vi "Save Last Print.vi"(8 "error in (no error)":errorcluster, 9 "Printing Date":string, 10 "SN":u32, 11 "Part Name":string) -> (0 "error out":errorcluster)   [LabVIEW 2017]
uses:
  <vilib>/Utility/config.llb/Write Key (U32).vi
  <vilib>/Utility/config.llb/Write Key (String).vi
  <vilib>/Utility/config.llb/NI_LVConfig.lvlib
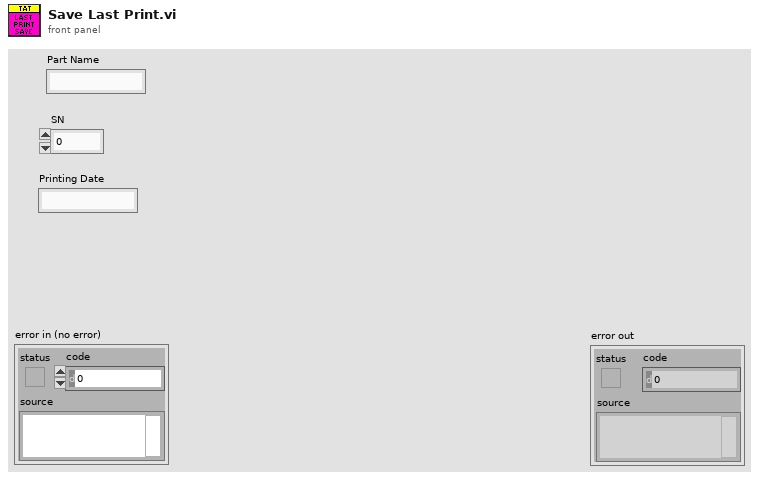
[diagram p1: front panel]
types:
  T1 = enum32{"invalid app kind", "Development System", "Run Time System", "Student Edition", "Embedded LabVIEW", "Evaluation", "Custom"}
  T2 = typedef "NI_LVConfig.lvlib/Config Data RefNum.ctl" = refnum<k1>
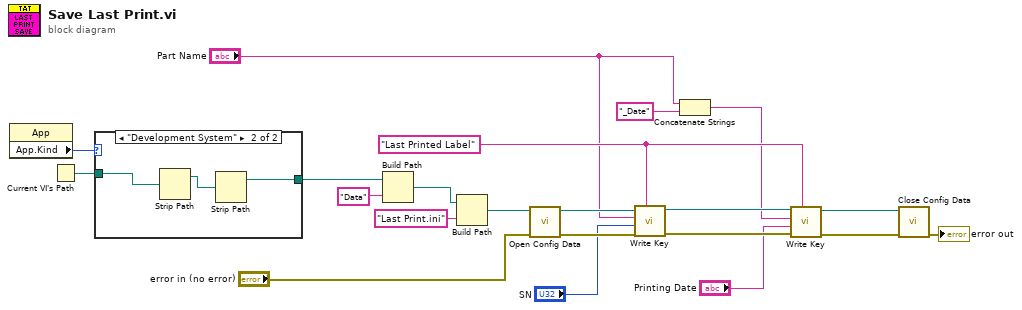
[diagram p0: block diagram]
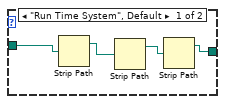
[diagram p2: hidden frame]
diagram:
  w7 = "Last Printed Label" ("section")
  n1 = property class="App"() -> ("App.Kind"=w20:T1)  [unwired: 2 in, 2 out]
  n2 = Current VI's Path() -> (path=w21:path)
  n3 = case shown="\"Development System\"" w20 {
    tunnel: w21 -> [w23 w27]
    tunnel: [w22 w26] -> w15
    frame "Run Time System", Default {
      n4 = Strip Path(path=w23) -> (stripped path=w25:path)  [unwired: 1 out]
      n5 = Strip Path(path=w25) -> (stripped path=w24:path)  [unwired: 1 out]
      n6 = Strip Path(path=w24) -> (stripped path=w22:path)  [unwired: 1 out]
    }
    frame "Development System" {
      n7 = Strip Path(path=w27) -> (stripped path=w28:path)  [unwired: 1 out]
      n8 = Strip Path(path=w28) -> (stripped path=w26:path)  [unwired: 1 out]
    }
  }
  n9 = Build Path(base path=w15, name or relative path="Data") -> (appended path=w18:path)
  n10 = Build Path(base path=w18, name or relative path="Last Print.ini") -> (appended path=w16:path)
  n11 = call <vilib>:"Open Config Data.vi"("error in (no error)"="error in (no error)", "configuration file path"=w16) -> ("error out"=w13:errorcluster, "refnum"=w10:T2)  [unwired: 7 in, 1 out]
  n12 = call-poly <vilib>:"Write Key.vi"("section"=w7, "error in (no error)"=w13, "value"="SN", "key"="Part Name", "refnum"=w10) -> ("error out"=w12:errorcluster, "refnum out"=w9:T2)  [unwired: 4 in, 1 out]
  n13 = Concatenate Strings("Part Name", "_Date" ("string")) -> (w4:string)
  n14 = call-poly <vilib>:"Write Key.vi"("section"=w7, "error in (no error)"=w12, "value"="Printing Date", "key"=w4, "refnum"=w9) -> ("error out"=w11:errorcluster, "refnum out"=w8:T2)  [unwired: 4 in, 1 out]
  n15 = call <vilib>:"Close Config Data.vi"("error in (no error)"=w11, "refnum"=w8) -> ("error out"=→"error out":errorcluster)  [unwired: 8 in, 1 out]
